vi "tables&columns.vi"(11 "选项":enum16{"初始化", "获取寄存器"}(ring)) -> (1 "columns":string[](array[string]), 3 "Tables&columns":T1)   [LabVIEW 2017]
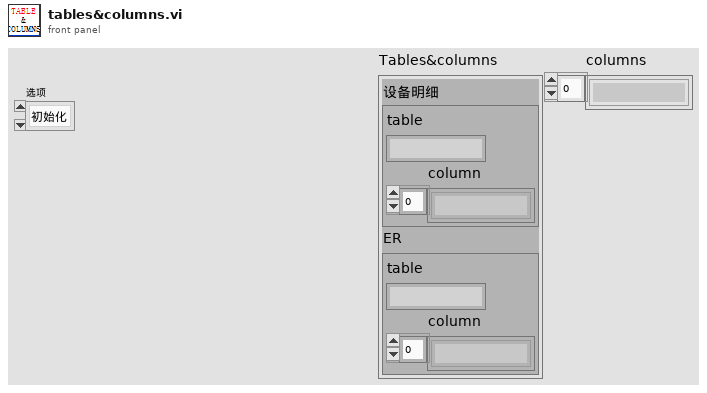
[diagram p1: front panel]
types:
  T1 = cluster{"设备明细":cluster{"table":string, "column":string[]}, "ER":cluster{"table":string, "column":string[]}}
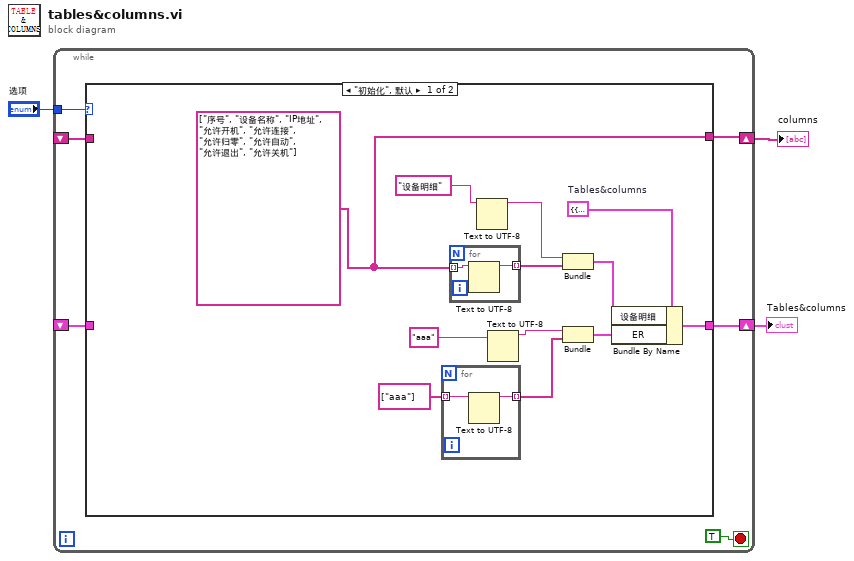
[diagram p0: block diagram]
diagram:
  n1 = while {
    tunnel: "选项" -> [w9]
    shift-right: [w8] -> w2
    shift-left: _ -> [w7]
    shift-right: [w5] -> w1
    shift-left: _ -> [w4]
    stop <- TRUE stop-if-true
    n2 = case shown="\"初始化\", 默认" w9 {
      tunnel: [w15 w27] -> w8
      tunnel: w7 -> [_ w27]
      tunnel: [w14 w26] -> w5
      tunnel: w4 -> [_ w26]
      frame "初始化", Default {
        w14 = string[] ["序号", "设备名称", "IP地址", "允许开机", "允许连接", "允许归零", "允许自动", "允许退出", "允许关机"] ("列首字符串[]")
        w21 = T1 {"设备明细"={"table"="", "column"=[]}, "ER"={"table"="", "column"=[]}}  # Tables&columns
        n3 = for {
          tunnel: string[] ["aaa"] ("all rows输出") -> [w25] mode=indexing
          tunnel: [w24] -> w18 mode=indexing
          n4 = Text to UTF-8(11:w25) -> (3:w24:string)  [unwired: 2 in, 1 out]
        }
        n5 = for {
          tunnel: w14 -> [w23] mode=indexing
          tunnel: [w22] -> w17 mode=indexing
          n6 = Text to UTF-8(11:w23) -> (3:w22:string)  [unwired: 2 in, 1 out]
        }
        n7 = Text to UTF-8(11:"设备明细") -> (3:w12:string)  [unwired: 2 in, 1 out]
        n8 = Text to UTF-8(11:"aaa") -> (3:w10:string)  [unwired: 2 in, 1 out]
        n9 = Bundle("utf-8 text"=w12, w17) -> (w20:cluster{"utf-8 text":string, string[]})  [unwired: 1 in]
        n10 = Bundle("utf-8 text"=w10, w18) -> (w19:cluster{"utf-8 text":string, string[]})  [unwired: 1 in]
        n11 = Bundle By Name(cluster=w21, "设备明细"=w20, "ER"=w19) -> (w15:T1)
      }
      frame "获取寄存器" {
      }
    }
  }
  "Tables&columns" <- w2
  "columns" <- w1
